vi "EEPROM UI MAIN.vi"(4 "error in (no error)":errorcluster, 5 "Path":path, 6 "Estyx device name":string, 7 "client ptr":u32) -> (0 "error out":errorcluster, 2 "EDGE/Rev String":string[](array[string]))   [LabVIEW 2010, in "lib1299.lvlib"]
doc: "This VI serves as the User Interface for programming the EEPROM on the EVM during testing. The EVM Name and EDGE numbers are read from EEPROM_EVM.ini and then the user can input the version of each item. The appropriate action can then be taken by selecting one of the two buttons at the bottom of the screen.\n\nInputs:\nclient ptr - reference to the estyx client\nEstyx device name - name of device (device directory in estyx)\nerror in - error input cluster\n\nOutputs:\n<PLL file configuration>\nEDGE/Rev ASCII Array - array of each element for programming the EEPROM converted to the appropriate ASCII numberic array.\nerror out - error output cluster"
uses:
  lib1299.lvlib
  Controls/EEPROM states.ctl
panel:
  in  "Stop":bool
  in  "Program":bool
  in  "BOM (assembly)":cluster{"EDGE Number":string, "Version":u16} {"Version" items=["A", "B", "C", "D", "E", "F", "G", "H", "I", "J", "K", "L", "M", "N", "O", "P", "Q", "R", "S", "T", "U", "V", "W", "X", "Y", "Z"]}
  out "EVM Name":string
  in  "PCA (assembly)":cluster{"EDGE Number":string, "Version":u16} {"Version" items=["A", "B", "C", "D", "E", "F", "G", "H", "I", "J", "K", "L", "M", "N", "O", "P", "Q", "R", "S", "T", "U", "V", "W", "X", "Y", "Z"]}
  in  "PWB (circuit board)":cluster{"EDGE Number":string, "Version":u16} {"Version" items=["A", "B", "C", "D", "E", "F", "G", "H", "I", "J", "K", "L", "M", "N", "O", "P", "Q", "R", "S", "T", "U", "V", "W", "X", "Y", "Z"]}
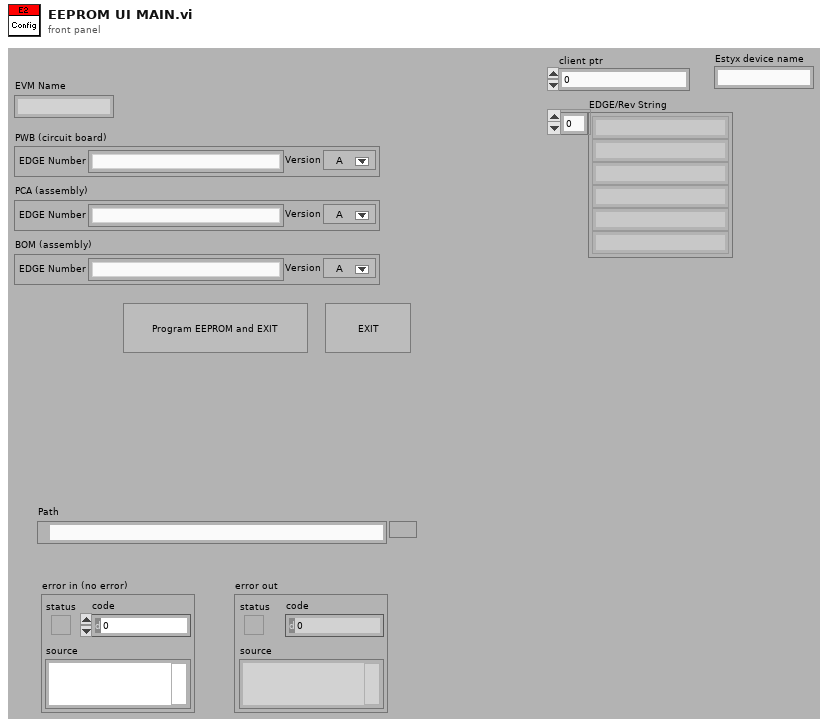
[diagram p1: front panel]
types:
  T1 = typedef "lib1299.lvlib/EEPROM states.ctl" = enum16{"Initialize", "Read INI", "User Input", "Add Date", "Write estyx", "Exit"}
  T2 = typedef "lib1299.lvlib/EEPROM_data.ctl" = cluster{"EVM Name":string, "PWB":T3, "PCA":T3, "BOM":T3}
  T3 = typedef "lib1299.lvlib/EDGE ITEM.ctl" = cluster{"EDGE No.":string, "Rev":u16}
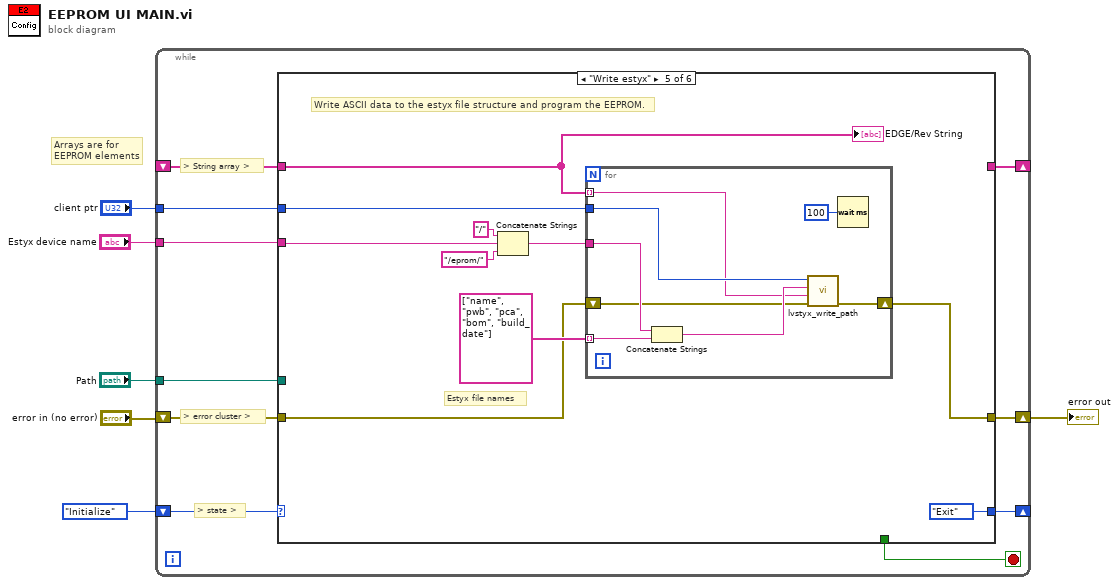
[diagram p0: block diagram]
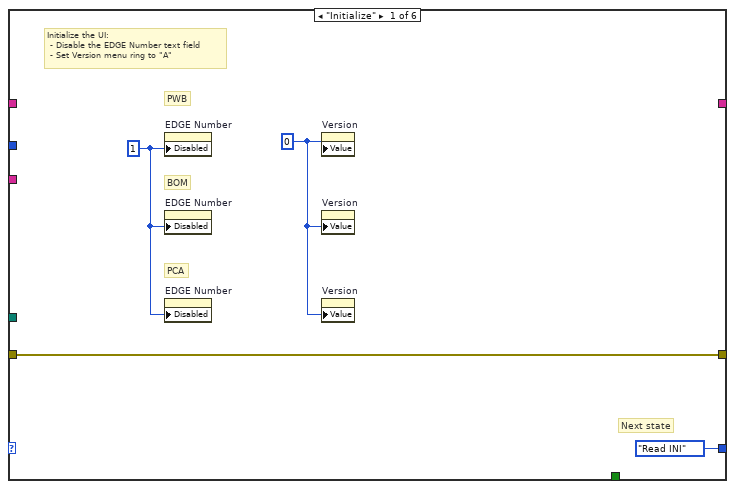
[diagram p2: hidden frame]
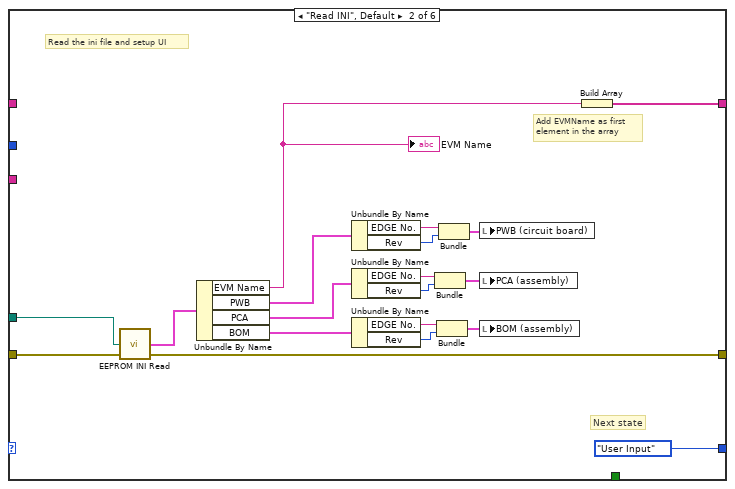
[diagram p3: hidden frame]
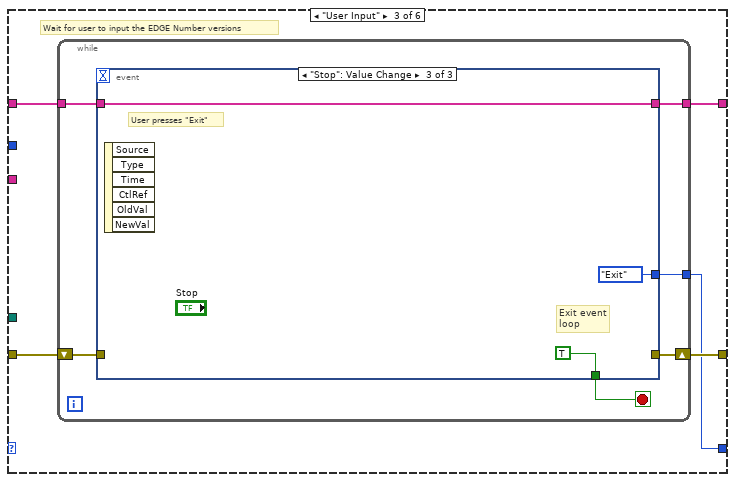
[diagram p4: hidden frame]
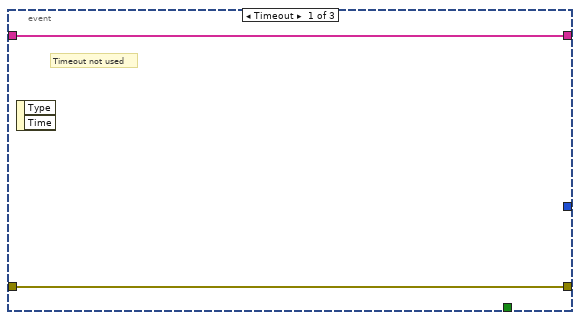
[diagram p5: hidden frame]
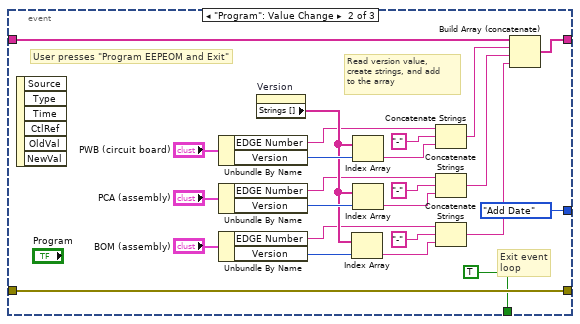
[diagram p6: hidden frame]
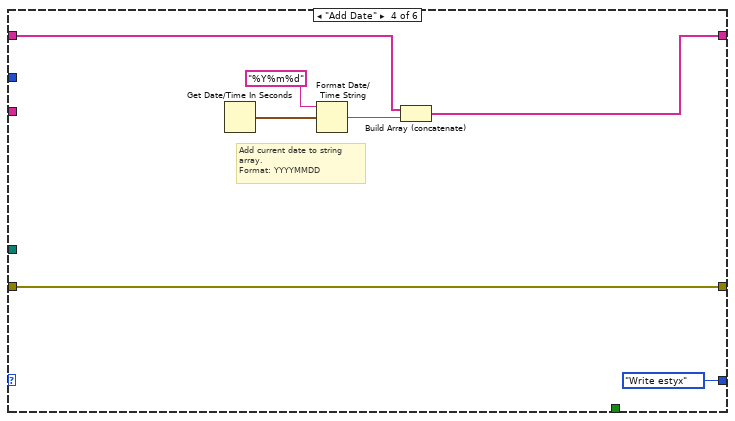
[diagram p7: hidden frame]
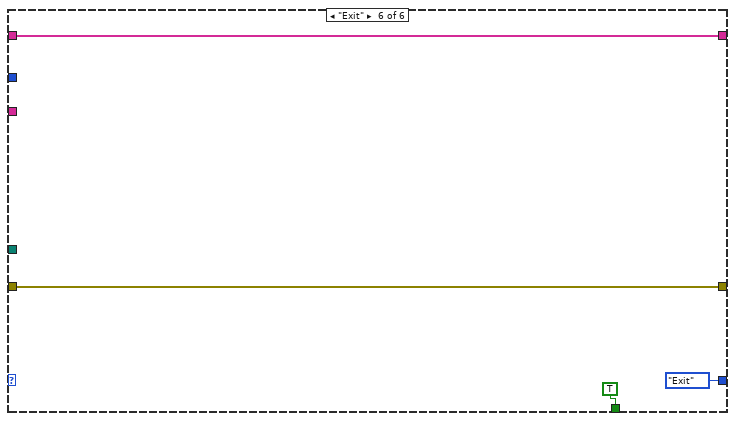
[diagram p8: hidden frame]
diagram:
  # "Arrays are for\nEEPROM elements"
  n1 = while {
    shift-right: [w13] -> _
    shift-left: EEPROM_states."Initialize" ("EEPROM states") -> [w16]
    shift-right: [w15] -> w3
    shift-left: "error in (no error)" -> [w14]
    shift-right: [w10] -> _
    shift-left: _ -> [w12]
    tunnel: "client ptr" -> [w9]
    tunnel: "Estyx device name" -> [w8]
    tunnel: "Path" -> [w7]
    stop <- w11 stop-if-true
    # "> state >"
    # "> error cluster >"
    # "> String array >"
    n2 = case shown="\"Write estyx\"" w16 {
      tunnel: w14 -> [w18 w39 w44 w86 w89 w106]
      tunnel: [w18 w38 w43 w86 w88 w106] -> w15
      tunnel: [EEPROM_states."Read INI" ("EEPROM states") EEPROM_states."User Input" ("EEPROM states") w40 EEPROM_states."Write estyx" ("EEPROM states") EEPROM_states."Exit" ("EEPROM states") EEPROM_states."Exit" ("EEPROM states")] -> w13
      tunnel: w12 -> [_ _ w42 w83 w87 w105]
      tunnel: [_ _ _ _ _ TRUE] -> w11
      tunnel: [_ w23 w41 w80 _ w105] -> w10
      tunnel: w9 -> [_ _ _ _ w90 _]
      tunnel: w8 -> [_ _ _ _ w95 _]
      tunnel: w7 -> [_ w21 _ _ _ _]
      frame "Initialize" {
        w20 = u8 1 ("Disabled")
        w17 = 0
        # "Next state"
        # "Initialize the UI:\n - Disable the EDGE Number text field\n - Set Version menu ring to \"A\""
        # "PCA"
        # "BOM"
        # "PWB"
        n3 = property on="EDGE Number" class="Str"("Disabled"=w20) -> ()  [unwired: 2 in, 2 out]
        n4 = property on="EDGE Number" class="Str"("Disabled"=w20) -> ()  [unwired: 2 in, 2 out]
        n5 = property on="EDGE Number" class="Str"("Disabled"=w20) -> ()  [unwired: 2 in, 2 out]
        n6 = property on="Version" class="Ring (strict)"("Value"=w17) -> ()  [unwired: 2 in, 2 out]
        n7 = property on="Version" class="Ring (strict)"("Value"=w17) -> ()  [unwired: 2 in, 2 out]
        n8 = property on="Version" class="Ring (strict)"("Value"=w17) -> ()  [unwired: 2 in, 2 out]
      }
      frame "Read INI", Default {
        # "Next state"
        # "Add EVMName as first\nelement in the array"
        # "Read the ini file and setup UI"
        n9 = call "EEPROM INI Read.vi"("error in (no error)"=w39, "Path"=w21) -> ("error out"=w38:errorcluster, "EEPROM Data"=w24:T2)  [unwired: 2 in]
        n10 = Unbundle By Name(w24) -> ("EVM Name"=w22:string, "PWB"=w36:T3, "PCA"=w26:T3, "BOM"=w25:T3)
        "EVM Name" <- w22
        n11 = Unbundle By Name(w36) -> ("EDGE No."=w35:string, "Rev"=w34:u16)
        n12 = Unbundle By Name(w26) -> ("EDGE No."=w31:string, "Rev"=w32:u16)
        n13 = Unbundle By Name(w25) -> ("EDGE No."=w29:string, "Rev"=w28:u16)
        n14 = Bundle("EDGE No."=w31, "Rev"=w32) -> (w30:cluster{"EDGE No.":string, "Rev":u16})  [unwired: 1 in]
        n15 = Bundle("EDGE No."=w29, "Rev"=w28) -> (w27:cluster{"EDGE No.":string, "Rev":u16})  [unwired: 1 in]
        n16 = Bundle("EDGE No."=w35, "Rev"=w34) -> (w33:cluster{"EDGE No.":string, "Rev":u16})  [unwired: 1 in]
        n17 = local write "PWB (circuit board)"(w33) -> ()
        n18 = local write "PCA (assembly)"(w30) -> ()
        n19 = local write "BOM (assembly)"(w27) -> ()
        n20 = Build Array(w22) -> (w23:string[])
      }
      frame "User Input" {
        # "Wait for user to input the EDGE Number versions"
        n21 = while {
          shift-right: [w49] -> w43
          shift-left: w44 -> [w50]
          tunnel: w42 -> [w47]
          tunnel: [w46] -> w41
          tunnel: [w45] -> w40
          stop <- w48 stop-if-true
          n22 = event shown="[2] \"Stop\": Value Change" {
            selector: _ -> [_ _ _]
            dyn-events: _ -> [_ _ _]
            timeout: _ -> [_ _ _]
            tunnel: w50 -> [w52 w76 _]
            tunnel: [w52 w76 _] -> w49
            tunnel: [_ TRUE TRUE] -> w48
            tunnel: w47 -> [w51 w62 w78]
            tunnel: [w51 w58 w78] -> w46
            tunnel: [_ EEPROM_states."Add Date" ("EEPROM states") EEPROM_states."Exit" ("EEPROM states")] -> w45
            event Timeout {
              # "Timeout not used"
              n23 = event-data() -> ()  [unwired: 1 in, 2 out]
            }
            event "Program": Value Change {
              # "Exit event\nloop"
              # "Read version value, \ncreate strings, and add\nto the array"
              # "User presses \"Program EEPEOM and Exit\""
              n24 = event-data() -> ()  [unwired: 1 in, 6 out]
              n25 = Unbundle By Name("PWB (circuit board)") -> ("EDGE Number"=w71:string, "Version"=w75:u16)
              n26 = Unbundle By Name("PCA (assembly)") -> ("EDGE Number"=w63:string, "Version"=w74:u16)
              n27 = Unbundle By Name("BOM (assembly)") -> ("EDGE Number"=w64:string, "Version"=w73:u16)
              n28 = property on="Version" class="Ring (strict)"() -> ("Strings []"=w72:string[])  [unwired: 2 in, 2 out]
              n29 = Index Array(array=w72, index=w73) -> (element=w65:string)
              n30 = Index Array(array=w72, index=w75) -> (element=w70:string)
              n31 = Index Array(array=w72, index=w74) -> (element=w66:string)
              n32 = Concatenate Strings(w71, "-" ("string"), w70) -> (w61:string)
              n33 = Concatenate Strings(w63, "-" ("string"), w66) -> (w60:string)
              n34 = Concatenate Strings(w64, "-" ("string"), w65) -> (w59:string)
              n35 = Build Array (concatenate)(w62, w61, w60, w59) -> (w58:string[])
            }
            event "Stop": Value Change {
              # "User presses \"Exit\""
              # "Exit event\nloop"
              n36 = event-data() -> ()  [unwired: 1 in, 6 out]
            }
          }
        }
      }
      frame "Add Date" {
        # "Add current date to string\narray.\nFormat: YYYYMMDD"
        n37 = Get Date/Time In Seconds() -> (seconds since 1Jan1904=w82:timestamp)
        n38 = Format Date/Time String(time format string (%c)="%Y%m%d", seconds (now)=w82) -> (date/time string=w84:string)  [unwired: 1 in]
        n39 = Build Array (concatenate)(w83, w84) -> (w80:string[])
      }
      frame "Write estyx" {
        # "Estyx file names"
        # "Write ASCII data to the estyx file structure and program the EEPROM."
        n40 = Concatenate Strings("/" ("string"), w95, "/eprom/" ("string")) -> (w92:string)
        n41 = for {
          tunnel: string[] ["name", "pwb", "pca", "bom", "build_date"] -> [w103] mode=indexing
          tunnel: w87 -> [w98] mode=indexing
          tunnel: w92 -> [w104]
          tunnel: w90 -> [w101]
          shift-right: [w99] -> w88
          shift-left: w89 -> [w100]
          n42 = Concatenate Strings(w104, w103) -> (w102:string)
          n43 = call "lvstyx_write_path.vi"("error in (no error)"=w100, "buf"=w98, "path"=w102, "client ptr"=w101) -> ("error out"=w99:errorcluster)  [unwired: 5 in, 2 out]
          n44 = Wait (ms)(milliseconds to wait=u32 100) -> ()  [unwired: 1 out]
        }
        "EDGE/Rev String" <- w87
      }
      frame "Exit" {
      }
    }
  }
  "error out" <- w3
